vi "reads_data.vi"(0 "Path":path, 5 "Key":string, 11 "error in (no error)":errorcluster) -> (4 "Value":string, 15 "error out":errorcluster)   [LabVIEW 2023]
uses:
  <vilib>/Utility/config.llb/Read Key (Double).vi
  <vilib>/Utility/config.llb/NI_LVConfig.lvlib
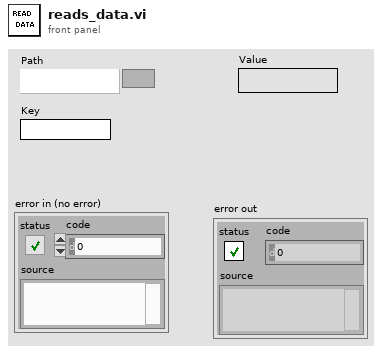
[diagram p1: front panel]
types:
  T1 = typedef "NI_LVConfig.lvlib/Config Data RefNum.ctl" = refnum<k1>
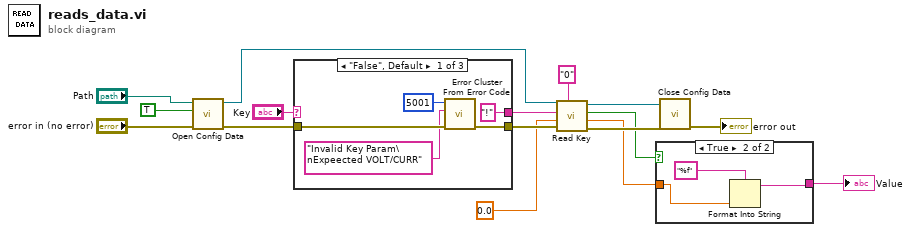
[diagram p0: block diagram]
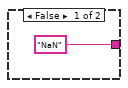
[diagram p2: hidden frame]
diagram:
  n1 = call <vilib>:"Open Config Data.vi"("error in (no error)"="error in (no error)", "create file if necessary (T)"=TRUE, "configuration file path"="Path") -> ("error out"=w6:errorcluster, "refnum"=w11:T1)  [unwired: 6 in, 1 out]
  n2 = case shown="\"False\", Default" "Key" {
    selector: "Key" -> [_ w23 w25]
    tunnel: ["!" w23 w25] -> w7
    tunnel: w6 -> [w21 w22 w24]
    tunnel: [w19 w22 w24] -> w5
    frame "False", Default {
      n3 = call <vilib>:"Error Cluster From Error Code.vi"("error in (no error)"=w21, "error message (\"\")"="Invalid Key Param\nExpeected VOLT/CURR" ("error message (\"\")"), "error code (0)"=5001) -> ("error out"=w19:errorcluster)  [unwired: 6 in]
    }
    frame "CURR" {
    }
    frame "VOLT" {
    }
  }
  n4 = call-poly <vilib>:"Read Key.vi"("section"="0", "error in (no error)"=w5, "default value"=0.0, "key"=w7, "refnum"=w11) -> ("error out"=w9:errorcluster, "value"=w2:dbl, "found?"=w3:bool, "refnum out"=w13:T1)  [unwired: 3 in]
  n5 = case shown="True" w3 {
    tunnel: ["NaN" w29] -> w1
    tunnel: w2 -> [_ w27]
    frame False {
    }
    frame True {
      n6 = Format Into String(format string="%f", w27) -> (resulting string=w29:string)  [unwired: 2 in, 1 out]
    }
  }
  "Value" <- w1
  n7 = call <vilib>:"Close Config Data.vi"("error in (no error)"=w9, "refnum"=w13) -> ("error out"=→"error out":errorcluster)  [unwired: 8 in, 1 out]
